vi "Set PS Settings.vi"(10 "PS_Settings In":T1[](array[typedef]), 11 "Array":refnum<visa-resource-name>[](array[refnum])) -> (3 "PS_Settings Out":T1[](array[typedef]))   [LabVIEW 2015]
uses:
  PS_Settings.ctl
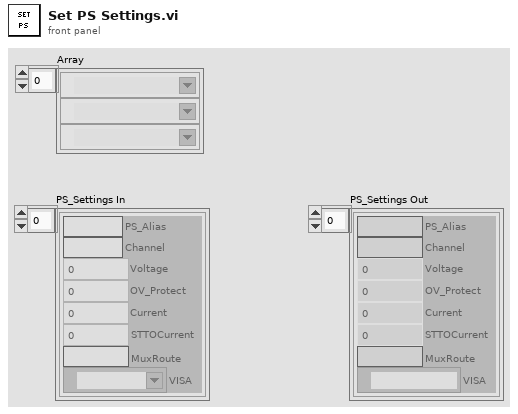
[diagram p1: front panel]
types:
  T1 = typedef "PS_Settings.ctl" = cluster{"PS_Alias":string, "Channel":string, "Voltage":dbl, "OV_Protect":dbl, "Current":dbl, "STTOCurrent":dbl, "MuxRoute":string, "VISA":refnum<visa-resource-name>}
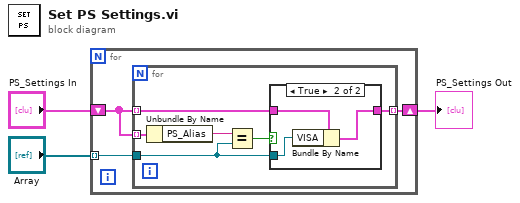
[diagram p0: block diagram]
diagram:
  n1 = for {
    tunnel: "Array" -> [w4] mode=indexing
    shift-right: [w5] -> w1
    shift-left: "PS_Settings In" -> [w6]
    n2 = for {
      tunnel: w6 -> [w12] mode=indexing
      tunnel: w6 -> [w8] mode=indexing
      tunnel: [w9] -> w5 mode=indexing
      tunnel: w4 -> [w7]
      n3 = Unbundle By Name(w12) -> ("PS_Alias"=w11:string)
      n4 = Equal?(x=w11, y=w7) -> (x = y?=w10:bool)
      n5 = case shown="True" w10 {
        tunnel: [w13 w15] -> w9
        tunnel: w8 -> [w13 w16]
        tunnel: w7 -> [_ w14]
        frame False {
        }
        frame True {
          n6 = Bundle By Name(cluster=w16, "VISA"=w14) -> (w15:T1)
        }
      }
    }
  }
  "PS_Settings Out" <- w1
